vi "c Spark Get Spark Model.vi"(8 "error in (no error)":errorcluster, 10 "c_Spark_SparkModel":T1 items=["c_Spark_Unknown", "c_Spark_SparkFlex", "c_Spark_SparkMax"], 11 "handle":T2) -> (0 "error out":errorcluster, 1 "function return":T3, 2 "c_Spark_SparkModel":T1 items=["c_Spark_Unknown", "c_Spark_SparkFlex", "c_Spark_SparkMax"], 3 "handle out":T2)   [LabVIEW 2023, in "REVLibDriver.lvlib"]
doc: "c_REVLib_ErrorCode c_Spark_GetSparkModel(c_Spark_handle handle,\n c_Spark_SparkModel* model);"
uses:
  REVLibDriver.lvlib
  home/systemcore/natinst/lib/libREVLibDriver.so
  Custom Controls/c_Spark_handle.ctl
  subvi/RevLibError.ctl
  Custom Controls/c_Spark_SparkModel.ctl
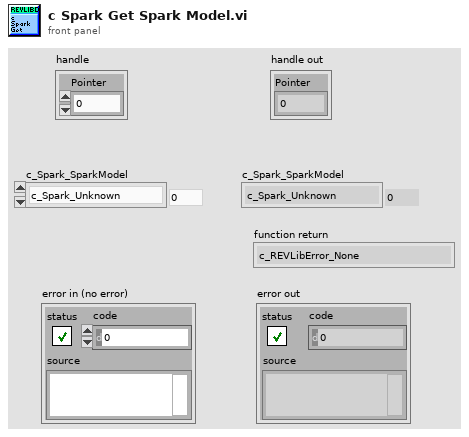
[diagram p1: front panel]
types:
  T1 = typedef "REVLibDriver.lvlib/c_Spark_SparkModel.ctl" = u16
  T2 = typedef "REVLibDriver.lvlib/c_Spark_handle.ctl" = cluster{"Pointer":u64}
  T3 = typedef "REVLibDriver.lvlib/RevLibError.ctl" = enum16{"c_REVLibError_None", "c_REVLibError_General", "c_REVLibError_CANTimeout", "c_REVLibError_NotImplemented", "c_REVLibError_HAL", "c_REVLibError_CantFindFirmware", "c_REVLibError_FirmwareTooOld", "c_REVLibError_FirmwareTooNew", "c_REVLibError_ParamInvalidID", "c_REVLibError_ParamMismatchType", "c_REVLibError_ParamAccessMode", "c_REVLibError_ParamInvalid", "c_REVLibError_ParamNotImplementedDeprecated", "c_REVLibError_FollowConfigMismatch", "c_REVLibError_Invalid", "c_REVLibError_SetpointOutOfRange", "c_REVLibError_Unknown", "c_REVLibError_CANDisconnected", "c_REVLibError_DuplicateCANId", "c_REVLibError_InvalidCANId", "c_REVLibError_SparkMaxDataPortAlreadyConfiguredDifferently", "c_REVLibError_SparkFlexBrushedWithoutDock", "c_REVLibError_InvalidBrushlessEncoderConfiguration", "c_REVLibError_FeedbackSensorIncompatibleWithDataPortConfig", "c_REVLibError_ParamInvalidChannel", "c_REVLibError_ParamInvalidValue", "c_REVLibError_CannotPersistParametersWhileEnabled", "c_REVLibError_NotReadyToReceiveCommand", "c_REVLibError_NumCodes"}
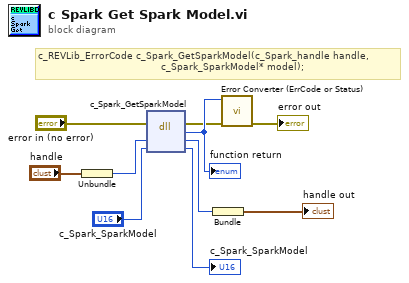
[diagram p0: block diagram]
diagram:
  # "c_REVLib_ErrorCode c_Spark_GetSparkModel(c_Spark_handle handle,\n                                         c_Spark_SparkModel* model);"
  n1 = Unbundle("handle") -> ("Pointer"=w2:u64)
  n2 = dll-call lib="home/systemcore/natinst/lib/libREVLibDriver.so" fn="c_Spark_GetSparkModel"(error in="error in (no error)", "handle"=w2, "model"="c_Spark_SparkModel") -> (error out=w4:errorcluster, "return type"=w10:u32, "handle"=w8:u64, "model"=→"c_Spark_SparkModel":u32)  [unwired: 2 in, 1 out]
  "function return" <- w10
  n3 = Bundle("handle"=w8) -> (→"handle out":cluster{"handle":u64})  [unwired: 1 in]
  n4 = call "Error Converter (ErrCode or Status).vi"("error in (no error)"=w4, "error code"=w10) -> ("error out"=→"error out":errorcluster)  [unwired: 9 in]
